vi "DeleteAndRefreshGraph(SubVI).vi"(6 "Legend":refnum<vi>, 7 "Lines":refnum<vi>, 8 "Error In":errorcluster, 9 "String in":string, 10 "Combo Box":refnum<vi>, 11 "XYGraph in":refnum<vi>) -> (0 "Error Out":errorcluster)   [LabVIEW 2018]
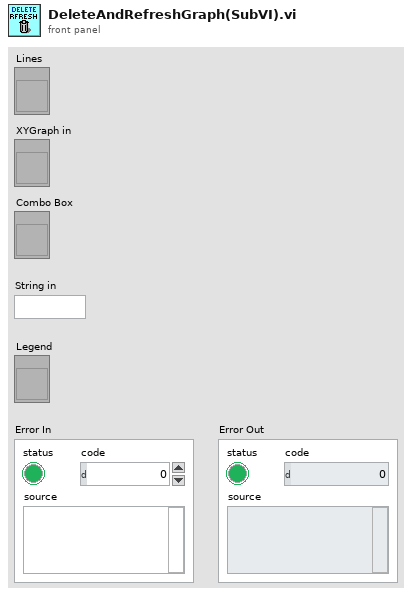
[diagram p1: front panel]
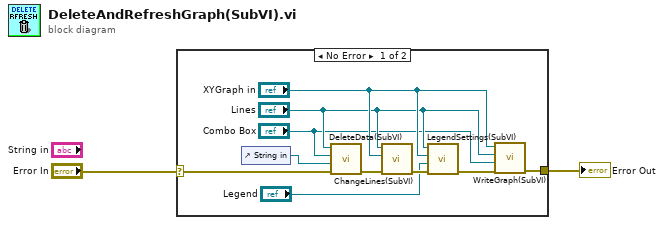
[diagram p0: block diagram]
diagram:
  n1 = case shown="No Error" "Error In" {
    selector: "Error In" -> [w6 w13]
    tunnel: [w5 w13] -> w1
    frame No Error {
      n2 = control-ref of="String in"() -> (w3:refnum<vi>)
      n3 = call "DeleteData(SubVI).vi"("Error In"=w6, "String in"=w3, "CmbBox Refnum"="Combo Box", "Array in"="Lines") -> ("Error Out"=w7:errorcluster)  [unwired: 7 in]
      n4 = call "ChangeLines(SubVI).vi"("Error In"=w7, "XYGraph Refnum"="XYGraph in", "Arr Refnum"="Lines") -> ("Error Out"=w9:errorcluster)  [unwired: 8 in]
      n5 = call "LegendSettings(SubVI).vi"("Error In"=w9, "Legend"="Legend", "XYGraph Refnum"="XYGraph in", "Arr Refnum"="Lines") -> ("Error Out"=w10:errorcluster)  [unwired: 7 in]
      n6 = call "WriteGraph(SubVI).vi"("Error In"=w10, "ComboBox in"="Combo Box", "Arr Refnum"="Lines", "XYGraph in"="XYGraph in") -> ("Error Out"=w5:errorcluster)  [unwired: 7 in]
    }
    frame Error {
    }
  }
  "Error Out" <- w1
